vi "GUI.vi"(8 "error in (no error)":errorcluster, 11 "object in":refnum<class "ExtraGUI.lvclass">) -> (0 "error out":errorcluster, 3 "object out":refnum<class "ExtraGUI.lvclass">)   [LabVIEW 2017, in "ExtraGUI.lvclass"]
uses:
  ExtraGUI.lvclass
  ExtraGUI.lvclass/ExtraGUI.ctl
panel:
  out "Appended Results":string
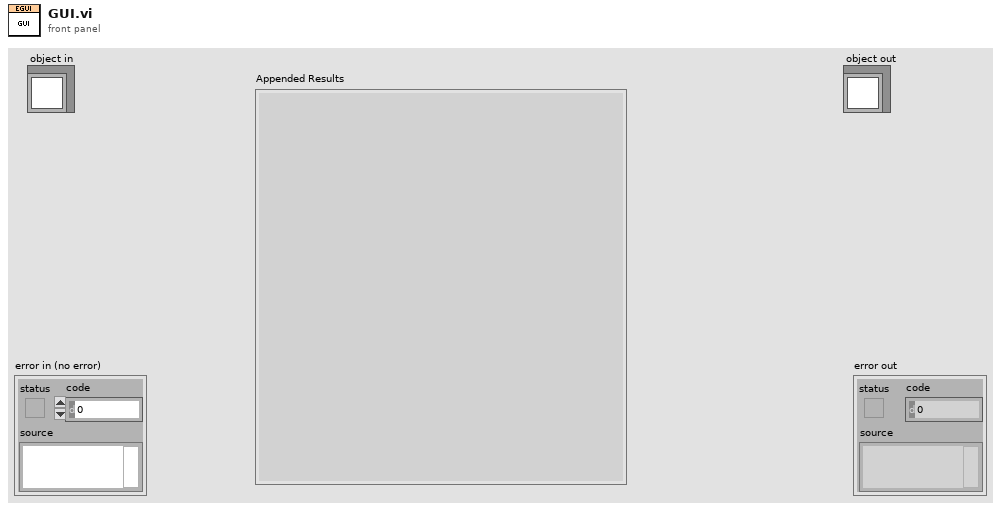
[diagram p1: front panel]
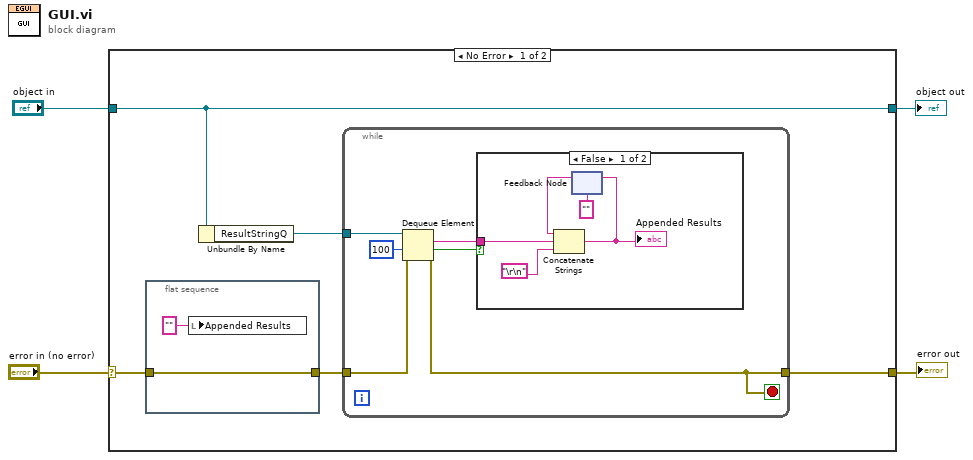
[diagram p0: block diagram]
diagram:
  n1 = case shown="No Error" "error in (no error)" {
    selector: "error in (no error)" -> [w6 w24]
    tunnel: [w7 w24] -> w3
    tunnel: [w9 w23] -> w1
    tunnel: "object in" -> [w9 w23]
    frame No Error {
      n2 = flat-sequence {
        tunnel: w6 -> [w10]
        tunnel: [w10] -> w5
        frame #0 {
          n3 = local write "Appended Results"("" ("Appended Results")) -> ()
        }
      }
      n4 = Unbundle By Name(w9) -> ("ResultStringQ"=w8:refnum<queue>)
      n5 = while {
        tunnel: w8 -> [w17]
        tunnel: w5 -> [w13]
        tunnel: [w12] -> w7
        stop <- w12 stop-if-true
        n6 = Dequeue Element(queue=w17, timeout in ms (-1)=100, error in (no error)=w13) -> (element=w15:string, timed out?=w16:bool, error out=w12:errorcluster)  [unwired: 1 out]
        n7 = case shown="False" w16 {
          tunnel: w15 -> [w22 _]
          frame False {
            n8 = feedback #1("") -> (w20:string)
            n9 = Concatenate Strings(w20, w22, "\r\n") -> (w19:string)
            "Appended Results" <- w19
            n10 = feedback-in #1(w19) -> ()
          }
          frame True {
          }
        }
      }
    }
    frame Error {
    }
  }
  "error out" <- w3
  "object out" <- w1
